vi "Apply Package Name to Enum Metadata.vi"(8 "error in":errorcluster, 10 "Package Name":string, 11 "gRPC Enum Metadata in":T1[](array[typedef])) -> (0 "error out":errorcluster, 3 "gRPC Enum Metadata out":T1[](array[typedef]))   [LabVIEW 2019, in "grpc-lvsupport.lvlib"]
uses:
  grpc-lvsupport.lvlib
  typeDefs/Enum Metadata.ctl
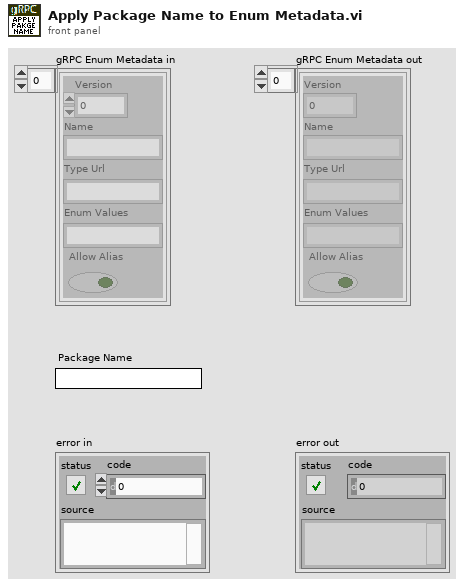
[diagram p1: front panel]
types:
  T1 = typedef "grpc-lvsupport.lvlib/Enum Metadata.ctl" = cluster{"Version":i32, "Name":string, "Type Url":string, "Enum Values":string, "Allow Alias":bool}
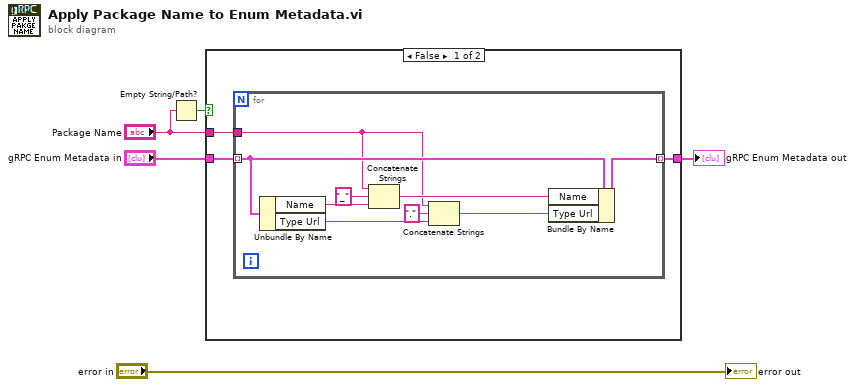
[diagram p0: block diagram]
diagram:
  n1 = Empty String/Path?(string/path="Package Name") -> (empty?=w3:bool)
  n2 = case shown="False" w3 {
    tunnel: "gRPC Enum Metadata in" -> [w8 w18]
    tunnel: [w7 w18] -> w1
    tunnel: "Package Name" -> [w6 _]
    frame False {
      n3 = for {
        tunnel: w8 -> [w13] mode=indexing
        tunnel: w6 -> [w9]
        tunnel: [w10] -> w7 mode=indexing
        n4 = Unbundle By Name(w13) -> ("Name"=w17:string, "Type Url"=w14:string)
        n5 = Concatenate Strings(w9, "_" ("string"), w17) -> (w12:string)
        n6 = Concatenate Strings(w9, "." ("string"), w14) -> (w11:string)
        n7 = Bundle By Name(cluster=w13, "Name"=w12, "Type Url"=w11) -> (w10:T1)
      }
    }
    frame True {
    }
  }
  "gRPC Enum Metadata out" <- w1
  "error out" <- "error in"
